vi "Receive Label Buffer with SDI Filter.vi"() -> ()   [LabVIEW 2019]
doc: "This program opens the specified card, configures the first receive channel from the configuration file with a filter for the label 206 message using FIFO List Buffering. Then the message data is continuously read and displayed based on received SDI setting."
uses:
  <instrlib>/BTICardLib/Private/Initialize By Card Number and Core Number.vi
  <instrlib>/BTICardLib/Private/Configure Core From XML.vi
  <instrlib>/BTI429Lib/Private/Rx/Configure/Configure Rx Channel From XML.vi
  <instrlib>/BTI429Lib/Private/Rx/Configure/Get Rx Label Handle Name.vi
  <instrlib>/BTI429Lib/Private/Core/Action-Status/Start Channel.vi
  <instrlib>/BTI429Lib/Private/Core/Action-Status/Stop Channel.vi
  <instrlib>/BTICardLib/BTICardLV.lvlib
  <instrlib>/BTI429Lib/BTI429LV.lvlib
panel:
  out "SDI11":u32[](array[numeric]) format="%08x"
  out "SDI10":u32[](array[numeric]) format="%08x"
  out "SDI01":u32[](array[numeric]) format="%08x"
  out "rx channel number":i32
  out "core number":i32
  out "error out":errorcluster
  in  "Channel Configuration XML file name":string="Channel Config - SDI.xml"
  in  "Core Configuration XML file name":string="Core Config.xml"
  in  "Card Number":i32
  out "SDI00":u32[](array[numeric]) format="%08x"
  in  "stop":bool
  # "ARINC 429: Receive Label Buffer with SDI Filter"
  # "©2016 Astronics Ballard Technology"
  # "This program opens the specified card, configures the first receive channel from the configuration file with a filter for the label 206 message using FIFO List Buffering. Then the message data is continuously read and displayed based on received SDI setting."
  # "Always Stop the card\nand Close the card when\ndone. Otherwise, the hardware\ncontinues to operate."
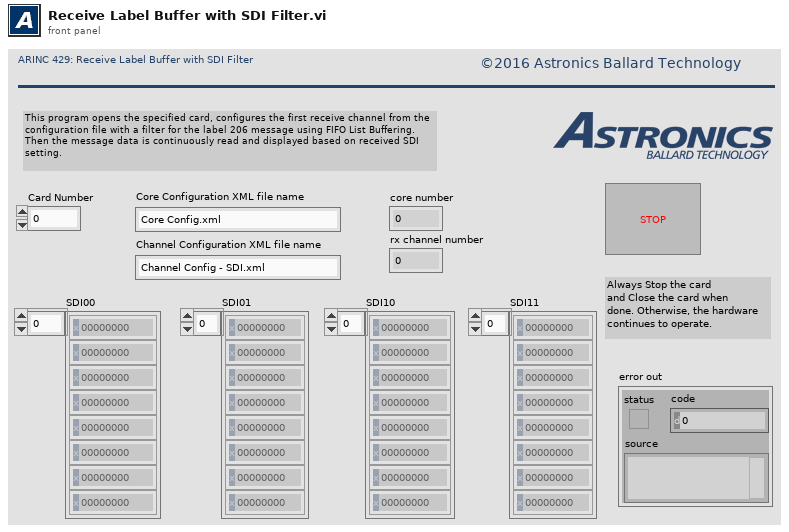
[diagram p1: front panel]
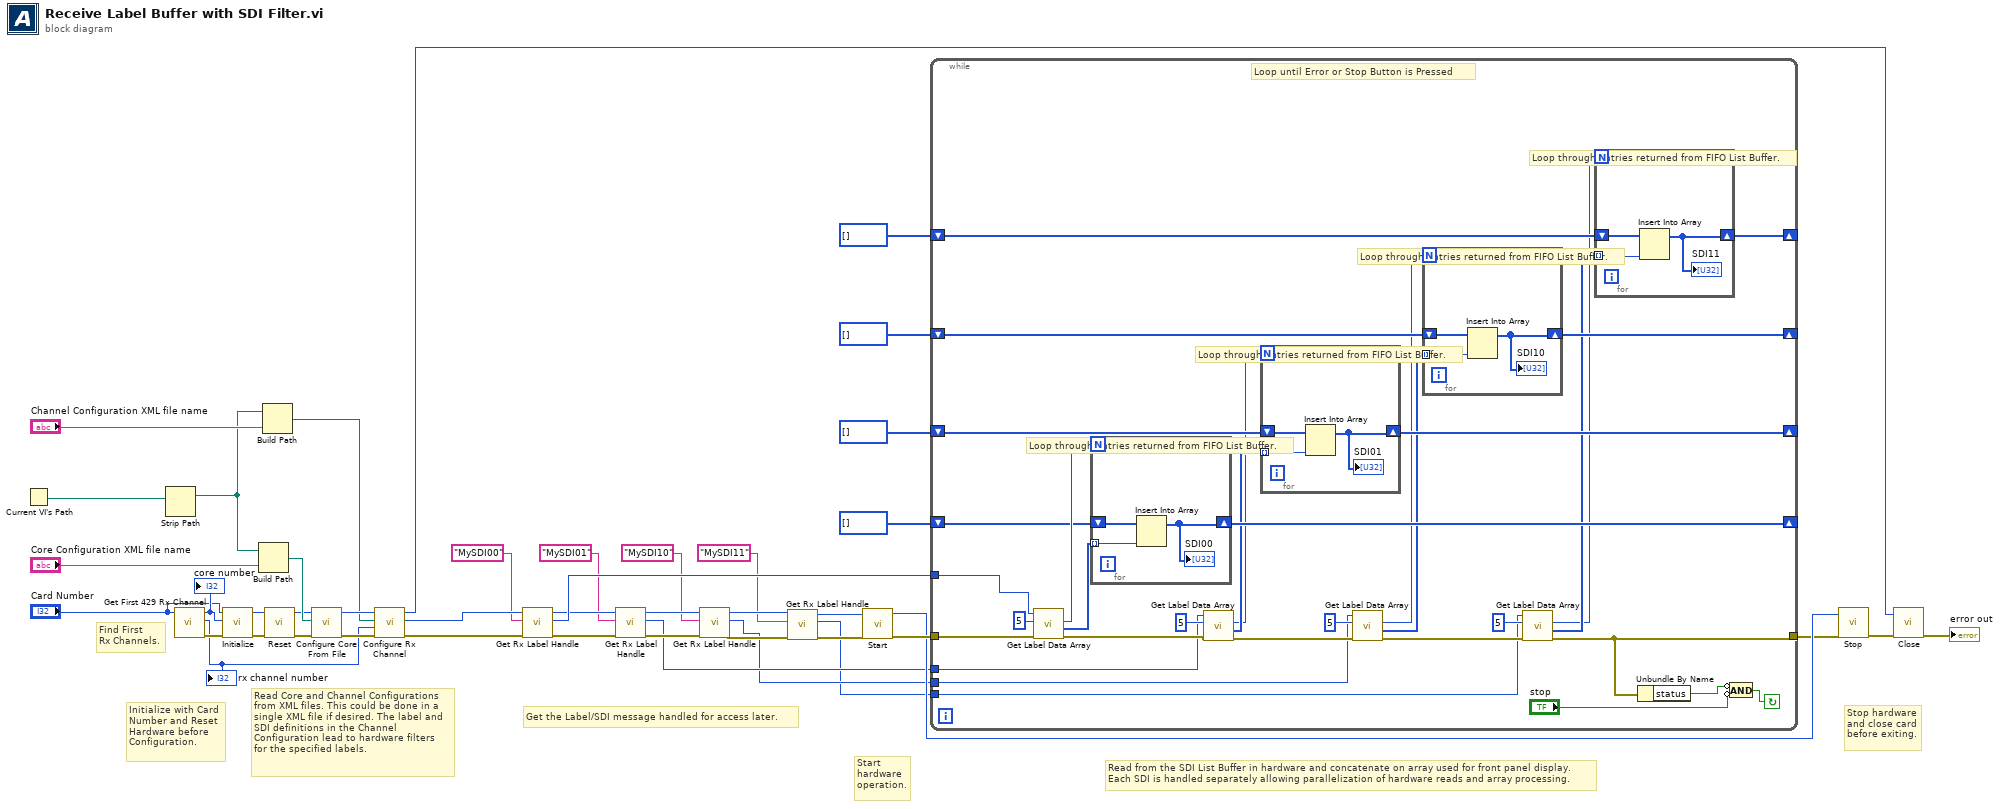
[diagram p0: block diagram]
diagram:
  # "Find First  \nRx Channels."
  # "Stop hardware\nand close card\nbefore exiting."
  # "Read from the SDI List Buffer in hardware and concatenate on array used for front panel display.\nEach SDI is handled separately allowing parallelization of hardware reads and array processing."
  # "Start\nhardware\noperation."
  # "Get the Label/SDI message handled for access later."
  # "Read Core and Channel Configurations\nfrom XML files. This could be done in a\nsingle XML file if desired. The label and\nSDI definitions in the Channel\nConfiguration lead to hardware filters\nfor the specified labels."
  # "Initialize with Card\nNumber and Reset\nHardware before\nConfiguration."
  n1 = Current VI's Path() -> (path=w34:path)
  n2 = Strip Path(path=w34) -> (stripped path=w31:path)  [unwired: 1 out]
  n3 = call "Get First 429 Rx Channel.vi"("Card Number"="Card Number") -> ("error out"=w24:errorcluster, "Channel Number"=w21:i32, "Core Number"=w23:i32)  [unwired: 8 in]
  "core number" <- w23
  "rx channel number" <- w21
  n4 = call-poly <instrlib>:"Initialize.vi"("error in (no error)"=w24, "core number"=w23, "card number"="Card Number") -> ("error out"=w25:errorcluster, "core handle out"=w28:u64)  [unwired: 7 in]
  n5 = Build Path(base path=w31, name or relative path="Core Configuration XML file name") -> (appended path=w29:path)
  n6 = Build Path(base path=w31, name or relative path="Channel Configuration XML file name") -> (appended path=w32:path)
  n7 = call <instrlib>:"Reset.vi"("error in (no error)"=w25, "core handle in"=w28) -> ("error out"=w26:errorcluster, "core handle out"=w27:u64)  [unwired: 8 in]
  n8 = call-poly <instrlib>:"Configure Core From File.vi"("error in (no error)"=w26, "configuration file path"=w29, "core handle in"=w27) -> ("error out"=w39:errorcluster, "core handle out"=w36:u64)  [unwired: 7 in]
  n9 = call-poly <instrlib>:"Configure Rx Channel.vi"("error in (no error)"=w39, "channel number in"=w21, "configuration file path"=w32, "core handle in"=w36) -> ("error out"=w16:errorcluster, "channel handle out"=w42:u64, "core handle out"=w15:u64)  [unwired: 5 in]
  n10 = call-poly <instrlib>:"Get Rx Label Handle.vi"("error in (no error)"=w16, "label name"="MySDI00", "channel handle in"=w42) -> ("error out"=w11:errorcluster, "label handle out"=w43:u64, "channel handle out"=w10:u64)  [unwired: 6 in]
  n11 = call-poly <instrlib>:"Get Rx Label Handle.vi"("error in (no error)"=w11, "label name"="MySDI01", "channel handle in"=w10) -> ("error out"=w12:errorcluster, "label handle out"=w3:u64, "channel handle out"=w9:u64)  [unwired: 6 in]
  n12 = call-poly <instrlib>:"Get Rx Label Handle.vi"("error in (no error)"=w12, "label name"="MySDI10", "channel handle in"=w9) -> ("error out"=w13:errorcluster, "label handle out"=w2:u64, "channel handle out"=w8:u64)  [unwired: 6 in]
  n13 = call-poly <instrlib>:"Get Rx Label Handle.vi"("error in (no error)"=w13, "label name"="MySDI11", "channel handle in"=w8) -> ("error out"=w14:errorcluster, "label handle out"=w1:u64, "channel handle out"=w7:u64)  [unwired: 6 in]
  n14 = call-poly <instrlib>:"Start.vi"("error in (no error)"=w14, "channel handle in"=w7) -> ("error out"=w44:errorcluster, "channel handle out"=w40:u64)  [unwired: 8 in]
  n15 = while {
    tunnel: w44 -> [w67]
    tunnel: w43 -> [w72]
    tunnel: [w48] -> w35
    shift-right: [w68] -> _
    shift-left: u32[] [] -> [w69]
    shift-right: [w64] -> _
    shift-left: u32[] [] -> [w63]
    shift-right: [w58] -> _
    shift-left: u32[] [] -> [w57]
    shift-right: [w52] -> _
    shift-left: u32[] [] -> [w51]
    tunnel: w3 -> [w47]
    tunnel: w2 -> [w46]
    tunnel: w1 -> [w45]
    stop <- w76 continue-if-true
    # "Loop until Error or Stop Button is Pressed"
    n16 = call <instrlib>:"Get Label Data Array.vi"("error in (no error)"=w67, "data items to read"=u32 5, "label handle in"=w72) -> ("error out"=w66:errorcluster, "data values"=w70:u32[], "data items read"=w71:u32)  [unwired: 5 in, 1 out]
    n17 = for {
      N: w71 -> [_]
      tunnel: w70 -> [w88] mode=indexing
      shift-right: [w86] -> w68
      shift-left: w69 -> [w87]
      # "Loop through entries returned from FIFO List Buffer."
      n18 = Insert Into Array(array=w87, new element=w88) -> (w86:u32[])  [unwired: 1 in]
      "SDI00" <- w86
    }
    n19 = call <instrlib>:"Get Label Data Array.vi"("error in (no error)"=w66, "data items to read"=u32 5, "label handle in"=w47) -> ("error out"=w59:errorcluster, "data values"=w62:u32[], "data items read"=w61:u32)  [unwired: 5 in, 1 out]
    n20 = for {
      N: w61 -> [_]
      tunnel: w62 -> [w85] mode=indexing
      shift-right: [w83] -> w64
      shift-left: w63 -> [w84]
      # "Loop through entries returned from FIFO List Buffer."
      n21 = Insert Into Array(array=w84, new element=w85) -> (w83:u32[])  [unwired: 1 in]
      "SDI01" <- w83
    }
    n22 = call <instrlib>:"Get Label Data Array.vi"("error in (no error)"=w59, "data items to read"=u32 5, "label handle in"=w46) -> ("error out"=w53:errorcluster, "data values"=w56:u32[], "data items read"=w55:u32)  [unwired: 5 in, 1 out]
    n23 = for {
      N: w55 -> [_]
      tunnel: w56 -> [w82] mode=indexing
      shift-right: [w80] -> w58
      shift-left: w57 -> [w81]
      # "Loop through entries returned from FIFO List Buffer."
      n24 = Insert Into Array(array=w81, new element=w82) -> (w80:u32[])  [unwired: 1 in]
      "SDI10" <- w80
    }
    n25 = call <instrlib>:"Get Label Data Array.vi"("error in (no error)"=w53, "data items to read"=u32 5, "label handle in"=w45) -> ("error out"=w48:errorcluster, "data values"=w50:u32[], "data items read"=w49:u32)  [unwired: 5 in, 1 out]
    n26 = for {
      N: w49 -> [_]
      tunnel: w50 -> [w79] mode=indexing
      shift-right: [w77] -> w52
      shift-left: w51 -> [w78]
      # "Loop through entries returned from FIFO List Buffer."
      n27 = Insert Into Array(array=w78, new element=w79) -> (w77:u32[])  [unwired: 1 in]
      "SDI11" <- w77
    }
    n28 = Unbundle By Name(w48) -> ("status"=w74:bool)
    n29 = Compound Arithmetic op=AND(invert w74, invert "stop") -> (w76:bool)
  }
  n30 = call-poly <instrlib>:"Stop.vi"("error in (no error)"=w35, "channel handle in"=w40) -> ("error out"=w41:errorcluster)  [unwired: 8 in, 1 out]
  n31 = call <instrlib>:"Close.vi"("error in (no error)"=w41, "core handle in"=w15) -> ("error out"=→"error out":errorcluster)  [unwired: 8 in, 1 out]
